vi "SimulatedDevice.vi"() -> ()   [LabVIEW 2017]
panel:
  in  "stop 2":bool
  in  "Boolean":bool
  out "Frequency 4":dbl
  out "Amplitude 2":dbl
  in  "Frequency 3":dbl=10.1 caption="Frequency"
  in  "Amplitude":dbl=1.0
  in  "Frequency 2":dbl=10.1 caption="Frequency"
  in  "Frequency":dbl=10.1
  out "Waveform Graph 2":dynamicdata(graph)
  out "Waveform Graph":dynamicdata(graph)
  in  "stop":bool
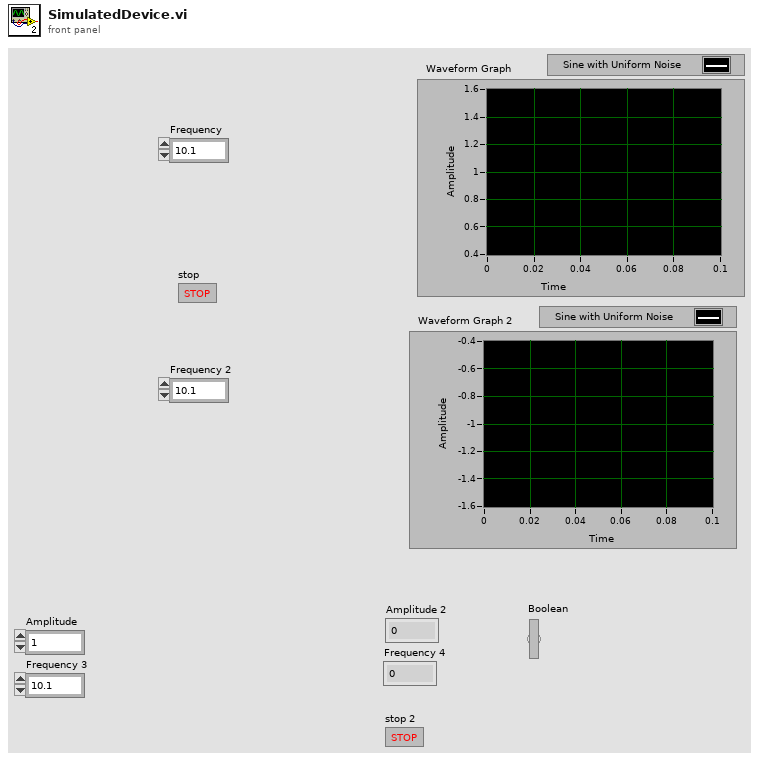
[diagram p1: front panel]
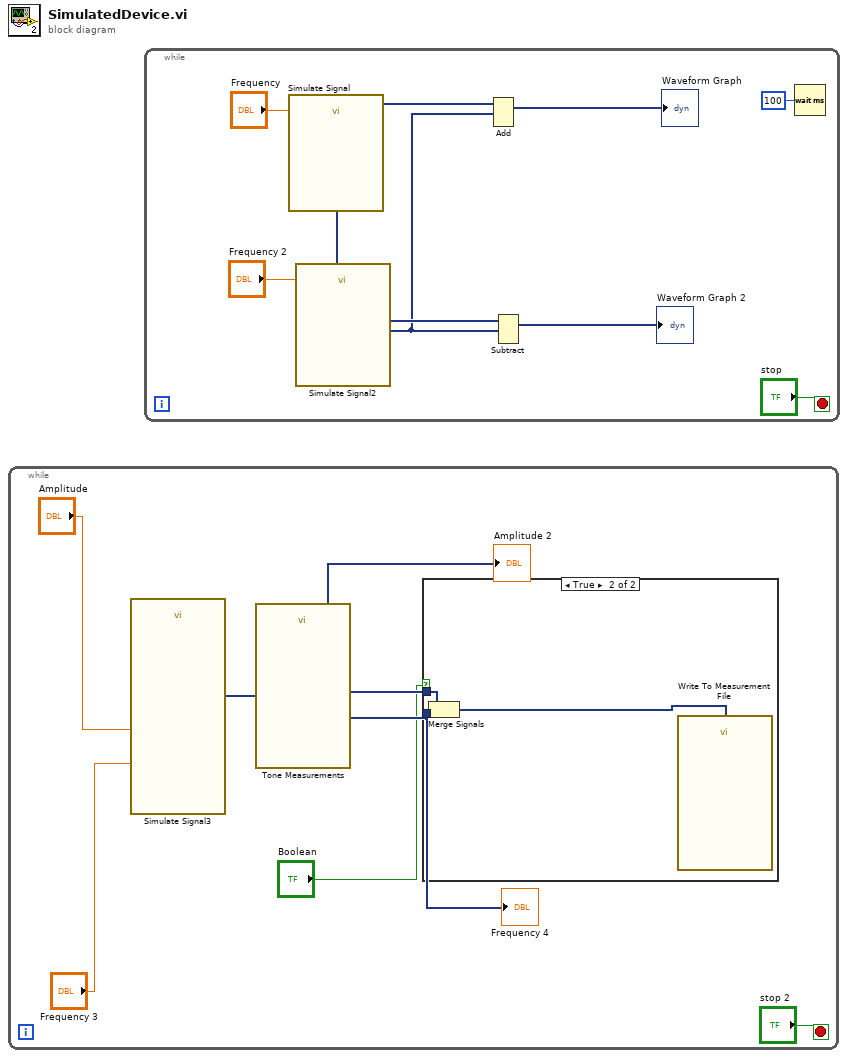
[diagram p0: block diagram]
diagram:
  n1 = while {
    stop <- "stop 2" stop-if-true
    n2 = call "Simulate Signal3"("Frequency"="Frequency 3", "Amplitude"="Amplitude") -> ("Sine"=w7:dynamicdata)  [unwired: 12 in, 1 out]
    n3 = call "Tone Measurements"("Signals"=w7) -> ("Frequency"=w3:dynamicdata, "Amplitude"=w4:dynamicdata)  [unwired: 8 in, 1 out]
    "Amplitude 2" <- w4
    "Frequency 4" <- w3
    n4 = case shown="True" "Boolean" {
      tunnel: w4 -> [_ w10]
      tunnel: w3 -> [_ w8]
      frame False {
      }
      frame True {
        n5 = Merge Signals(w10, w8) -> (w9:dynamicdata)
        n6 = call "Write To Measurement File"("Signals"=w9) -> ()  [unwired: 16 in, 3 out]
      }
    }
  }
  n7 = while {
    stop <- "stop" stop-if-true
    n8 = call "Simulate Signal"("Frequency"="Frequency") -> ("Sine with Uniform Noise"=w17:dynamicdata)  [unwired: 13 in, 1 out]
    n9 = call "Simulate Signal2"("Frequency"="Frequency 2") -> ("Square"=w16:dynamicdata)  [unwired: 13 in, 1 out]
    n10 = Add(1:w16, 2:w17) -> (0:→"Waveform Graph":dynamicdata)  [unwired: 1 in, 1 out]
    n11 = Subtract(1:w16, 2:w17) -> (0:→"Waveform Graph 2":dynamicdata)  [unwired: 1 in, 1 out]
    n12 = Wait (ms)(milliseconds to wait=u32 100) -> ()  [unwired: 1 out]
  }
